vi "HexformatToASCII.vi"() -> ()   [LabVIEW 2018]
panel:
  out "String(real ASCII) normal display":string
  out "String(real ASCII) '\\'codes display":string
  out "String(real ASCII) Hex display":string
  in  "String (HEX formatted ASCII)":string="09124E4F21CD0024FFFFFFFFFFFFFFFF"
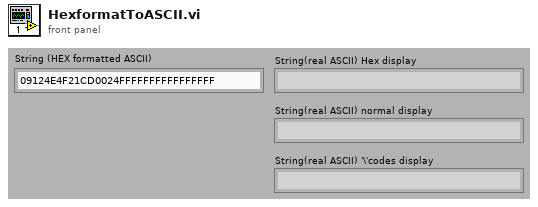
[diagram p1: front panel]
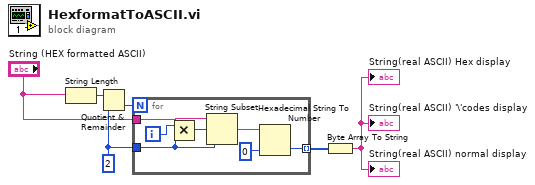
[diagram p0: block diagram]
diagram:
  w3 = 2 ("y")
  n1 = String Length(string="String (HEX formatted ASCII)") -> (length=w5:i32)
  n2 = Quotient & Remainder(x=w5, y=w3) -> (floor(x/y)=w4:i32)  [unwired: 1 out]
  n3 = for {
    N: w4 -> [_]
    tunnel: "String (HEX formatted ASCII)" -> [w11]
    tunnel: [w12] -> w6 mode=indexing
    tunnel: w3 -> [w7]
    i -> [w8]
    n4 = Multiply(x=w8, y=w7) -> (x*y=w9:i32)
    n5 = String Subset(string=w11, offset (0)=w9, length (rest)=w7) -> (substring=w10:string)
    n6 = Hexadecimal String To Number(string=w10, default (0uL)=u8 0) -> (number=w12:u8)  [unwired: 1 in, 1 out]
  }
  n7 = Byte Array To String(unsigned byte array=w6) -> (string=→"String(real ASCII) Hex display" →"String(real ASCII) '\\'codes display" →"String(real ASCII) normal display":string)
